vi "Inverse Step 4 (SubVI).vi"(0 "lblc":dbl, 1 "rbrc":dbl, 2 "aLB":dbl, 3 "aRB":dbl, 4 "aLB1":dbl, 5 "aRB1":dbl, 6 "aLB2":dbl, 7 "aRB2":dbl) -> (20 "lcx2":dbl, 21 "lcy2":dbl, 22 "rcx2":dbl, 23 "rcy2":dbl, 24 "aLB-aLB2":dbl, 25 "aRB-aRB2":dbl)   [LabVIEW 2015]
uses:
  <vilib>/express/express arith-compare/Formula/XNode/ExpressFormulaBlockNode.xnode
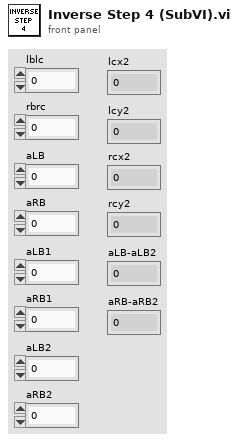
[diagram p1: front panel]
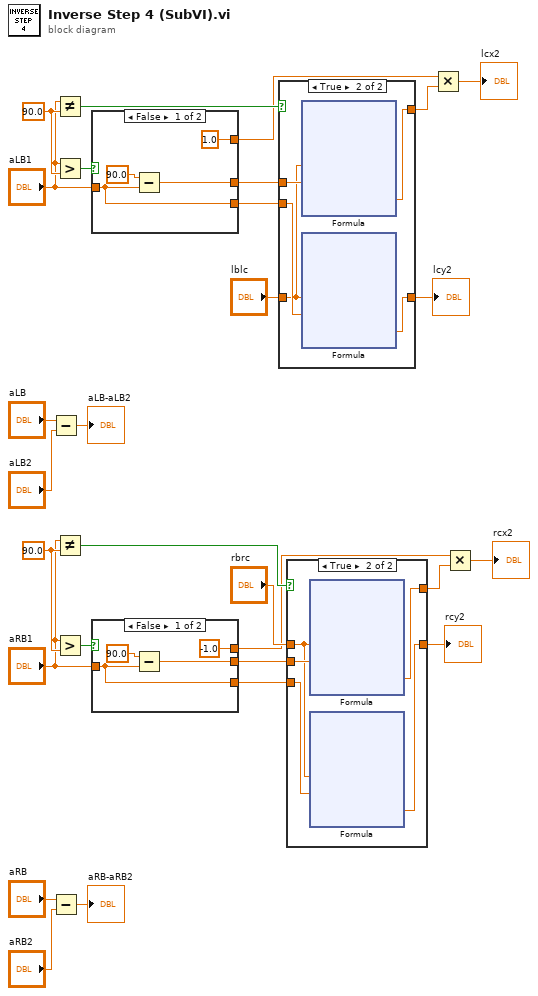
[diagram p0: block diagram]
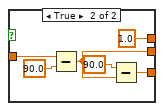
[diagram p2: hidden frame]
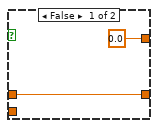
[diagram p3: hidden frame]
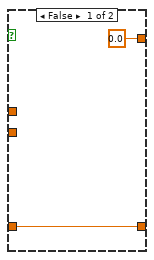
[diagram p4: hidden frame]
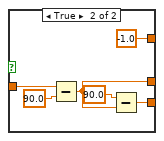
[diagram p5: hidden frame]
diagram:
  w20 = 90.0 ("y")
  w21 = 90.0 ("y")
  n1 = Subtract(x="aLB", y="aLB2") -> (x-y=→"aLB-aLB2":dbl)
  n2 = Subtract(x="aRB", y="aRB2") -> (x-y=→"aRB-aRB2":dbl)
  n3 = Not Equal?(x="aLB1", y=w21) -> (x != y?=w23:bool)
  n4 = Greater?(x="aLB1", y=w21) -> (0:w24:bool)
  n5 = Not Equal?(x="aRB1", y=w20) -> (x != y?=w22:bool)
  n6 = Greater?(x="aRB1", y=w20) -> (0:w9:bool)
  n7 = case shown="False" w24 {
    tunnel: "aLB1" -> [w30 w38]
    tunnel: [w31 w35] -> w18
    tunnel: [w30 w34] -> w19
    tunnel: [1.0 -1.0] -> w14
    frame False {
      n8 = Subtract(x=90.0, y=w30) -> (x-y=w31:dbl)
    }
    frame True {
      n9 = Subtract(x=w38, y=90.0) -> (x-y=w35:dbl)
      n10 = Subtract(x=90.0, y=w35) -> (x-y=w34:dbl)
    }
  }
  n11 = case shown="False" w9 {
    tunnel: "aRB1" -> [w40 w48]
    tunnel: [w41 w45] -> w16
    tunnel: [w40 w44] -> w17
    tunnel: [-1.0 1.0] -> w11
    frame False {
      n12 = Subtract(x=90.0, y=w40) -> (x-y=w41:dbl)
    }
    frame True {
      n13 = Subtract(x=w48, y=90.0) -> (x-y=w45:dbl)
      n14 = Subtract(x=90.0, y=w45) -> (x-y=w44:dbl)
    }
  }
  n15 = case shown="True" w23 {
    tunnel: w19 -> [_ w55]
    tunnel: w18 -> [_ w54]
    tunnel: [0.0 ("Result") w53] -> w15
    tunnel: [w50 w52] -> w1
    tunnel: "lblc" -> [w50 w51]
    frame False {
    }
    frame True {
      n16 = xnode "Formula"("lbrc"=w51, "aRX"=w54) -> ("Result"=w53:dbl)  [unwired: 1 in, 1 out]
      n17 = xnode "Formula"("lbrc"=w51, "aRY"=w55) -> ("Result"=w52:dbl)  [unwired: 1 in, 1 out]
    }
  }
  "lcy2" <- w1
  n18 = case shown="True" w22 {
    tunnel: w17 -> [_ w82]
    tunnel: w16 -> [_ w81]
    tunnel: [0.0 ("Result") w80] -> w10
    tunnel: [w77 w79] -> w2
    tunnel: "rbrc" -> [w77 w78]
    frame False {
    }
    frame True {
      n19 = xnode "Formula"("rblc"=w78, "aLX"=w81) -> ("Result"=w80:dbl)  [unwired: 1 in, 1 out]
      n20 = xnode "Formula"("rblc"=w78, "aLY"=w82) -> ("Result"=w79:dbl)  [unwired: 1 in, 1 out]
    }
  }
  "rcy2" <- w2
  n21 = Multiply(x=w14, y=w15) -> (x*y=→"lcx2":dbl)
  n22 = Multiply(x=w11, y=w10) -> (x*y=→"rcx2":dbl)
